vi "Sound_gen4.vi"(0 "Frequency":dbl, 2 "Sound time(s)":dbl=1.0, 4 "Dit time(ms)":u32, 10 "Volume":dbl(knob) scale=0.0..100.0, 11 "stop":bool, 13 "task ID":T1 format="%.0x", 14 "Is space":bool, 15 "error in (no error)":errorcluster) -> (6 "Sound On/Off":bool=TRUE, 22 "task ID out":T1 format="%.0x")   [LabVIEW 2022 SP3]
uses:
  <vilib>/sound2/lvsound2.llb/Sound Output Task ID.ctl
  <vilib>/sound2/lvsound2.llb/Sound Output Set Volume (Single).vi
  <vilib>/sound2/lvsound2.llb/Sound Output Write (DBL Single).vi
panel:
  out "error out":errorcluster
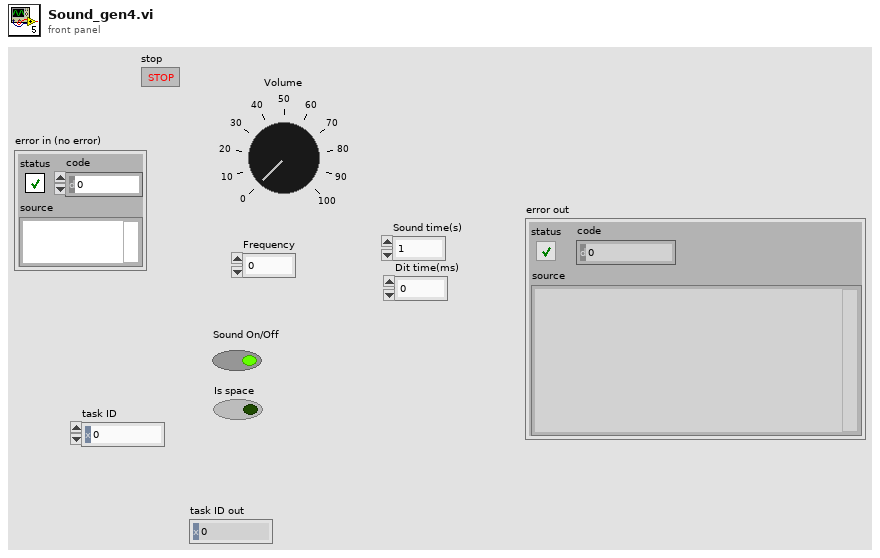
[diagram p1: front panel]
types:
  T1 = typedef "Sound Output Task ID.ctl" = u32
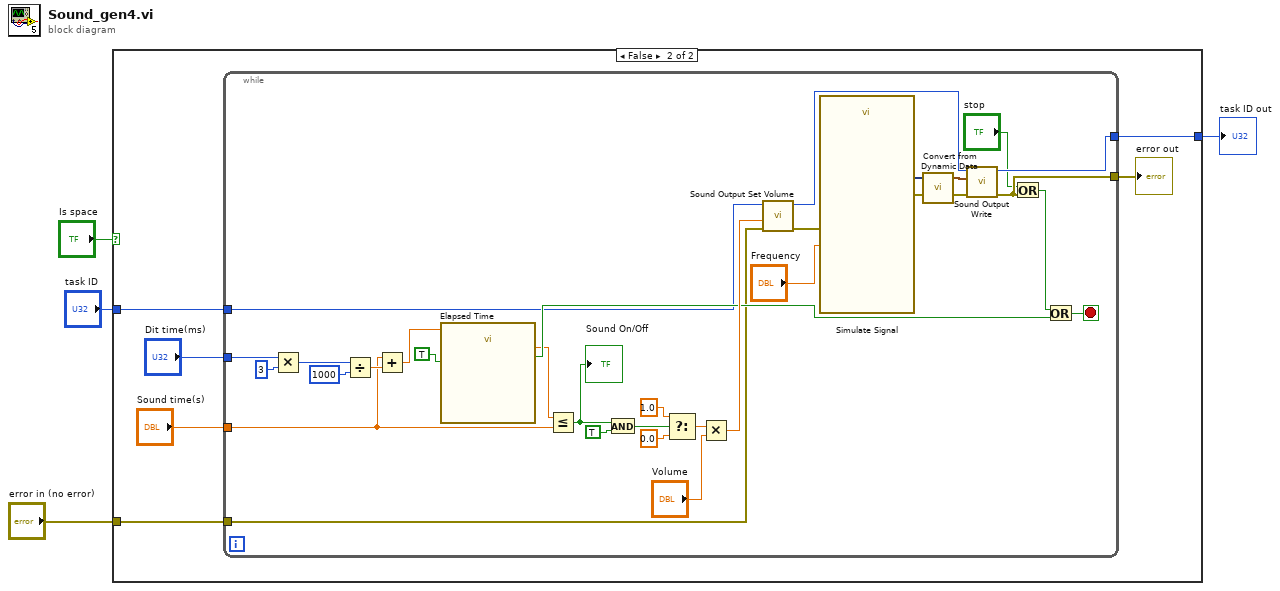
[diagram p0: block diagram]
diagram:
  n1 = case shown="False" "Is space" {
    tunnel: [w5 w8] -> w1
    tunnel: "error in (no error)" -> [_ w7]
    tunnel: "task ID" -> [w5 w6]
    frame True {
      # "space"
    }
    frame False {
      n2 = while {
        tunnel: [w41] -> w8
        tunnel: [w42] -> w9
        tunnel: "Sound time(s)" -> [w15]
        tunnel: "Dit time(ms)" -> [w23]
        tunnel: w7 -> [w14]
        tunnel: w6 -> [w13]
        stop <- w24 stop-if-true
        n3 = Multiply(x=w23, y=u32 3) -> (x*y=w18:u32)
        n4 = Divide(x=w18, y=u32 1000 ("x")) -> (x/y=w16:dbl)
        n5 = Add(x=w15, y=w16) -> (x+y=w20:dbl)
        n6 = call "Elapsed Time"("Time Target (s)"=w20, "Auto Reset"=TRUE) -> ("Elapsed Time (s)"=w19:dbl, "Time has Elapsed"=w21:bool)  [unwired: 10 in, 6 out]
        n7 = Less Or Equal?(x=w19, y=w15) -> (x <= y?=w12:bool)
        "Sound On/Off" <- w12
        n8 = And(x=w12, y=TRUE) -> (x .and. y?=w33:bool)
        n9 = Select(t=1.0, s=w33, f=0.0) -> (s? t:f=w29:dbl)
        n10 = Multiply(x=w29, y="Volume") -> (x*y=w28:dbl)
        n11 = call-poly <vilib>:"Sound Output Set Volume.vi"("error in (no error)"=w14, "volume"=w28, "task ID"=w13) -> ("error out"=w39:errorcluster, "task ID out"=w37:T1)  [unwired: 7 in]
        n12 = call "Simulate Signal"("Frequency"="Frequency", "error in (no error)"=w39) -> ("Sine"=w38:dynamicdata, "error out"=w35:errorcluster)  [unwired: 12 in]
        n13 = call "Convert from Dynamic Data"("Dynamic Data Type"=w38) -> ("Waveform"=w36:waveform(dbl))  [unwired: 3 in]
        n14 = call-poly <vilib>:"Sound Output Write.vi"("error in (no error)"=w35, "data"=w36, "task ID"=w37) -> ("error out"=w42:errorcluster, "task ID out"=w41:T1)  [unwired: 7 in]
        n15 = Or(x="stop", y=w42) -> (x .or. y?=w25:bool)
        n16 = Or(x=w25, y=w21) -> (x .or. y?=w24:bool)
      }
      "error out" <- w9
    }
  }
  "task ID out" <- w1
